vi "Log Initialization Results.vi"(8 "error in":errorcluster, 9 "Values":variant, 10 "Instrument":string, 11 "TDMS in":refnum<class "TDMS.lvclass">) -> (0 "error out":errorcluster, 3 "TDMS out":refnum<class "TDMS.lvclass">)   [LabVIEW 2019, in "TDMS.lvlib" / "TDMS.lvclass"]
uses:
  TDMS.lvclass
  builds/Tools/Report.lvlibp/Custom Controls/Report Action.ctl
  builds/Tools/Report.lvlibp/Report.lvclass
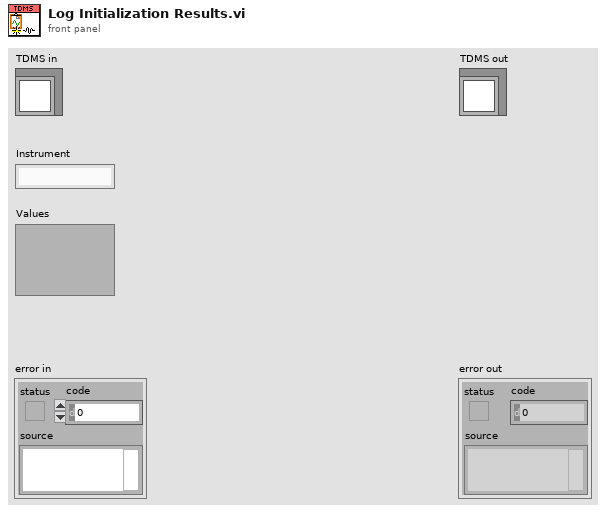
[diagram p1: front panel]
types:
  T1 = typedef "Report.lvlibp/Report.lvclass/Report Action.ctl" = enum16{"Create", "Append", "Destroy"}
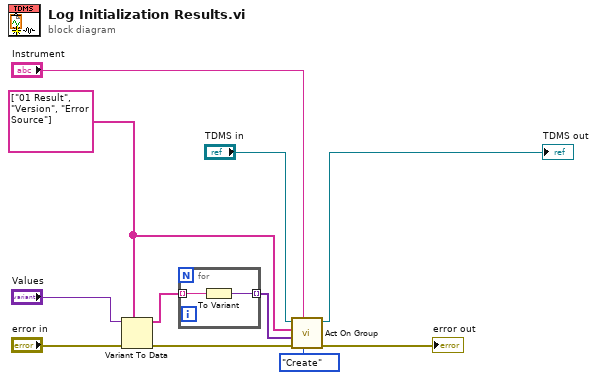
[diagram p0: block diagram]
diagram:
  w1 = string[] ["01 Result", "Version", "Error Source"]
  n1 = Variant To Data(error in="error in", type=w1, Variant="Values") -> (data=w5:string[], error out=w4:errorcluster)
  n2 = for {
    tunnel: w5 -> [w13] mode=indexing
    tunnel: [w12] -> w2 mode=indexing
    n3 = To Variant(anything=w13) -> (Variant=w12:variant)
  }
  n4 = call-dynamic "Act On Group.vi"("Report Action"=Report_Action."Create", "Group Name"="Instrument", "error in"=w4, "Values"=w2, "Parameters"=w1, "TDMS in"="TDMS in") -> ("error out"=→"error out":errorcluster, "TDMS out"=→"TDMS out":refnum<class "TDMS.lvclass">)  [unwired: 4 in]
